vi "Estimate Time.vi"(8 "error in (no error)":errorcluster, 11 "Scan Driver in":refnum<class "Scan Driver.lvclass">) -> (0 "error out":errorcluster, 1 "Seconds":dbl[unit], 2 "Time Estimate":string, 3 "Scan Driver out":refnum<class "Scan Driver.lvclass">)   [LabVIEW 2009, in "Scan Driver.lvclass"]
doc: "Estimate the time needed to complete this Scan Driver instance, using data from member Scanner and Reader."
uses:
  Scan Driver.lvclass
  Scan Driver.lvclass/Scan Driver.ctl
  Readers/Reader/Reader.lvclass
  Scanners/Scanner/Scanner.lvclass
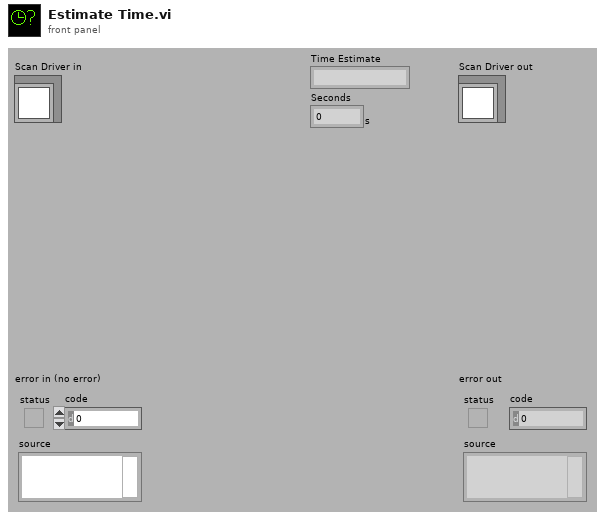
[diagram p1: front panel]
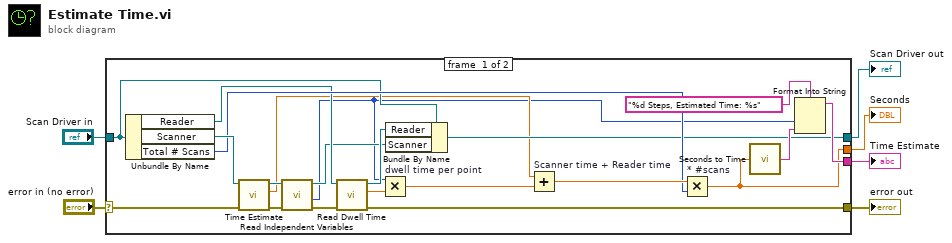
[diagram p0: block diagram]
diagram:
  n1 = case shown="No Error" "error in (no error)" {
    selector: "error in (no error)" -> [w10 w29]
    tunnel: [w23 _] -> w2
    tunnel: [w22 _] -> w1
    tunnel: [w14 w28] -> w5
    tunnel: [w8 w29] -> w6
    tunnel: "Scan Driver in" -> [w13 w28]
    frame #0 {
      n2 = Unbundle By Name(w13) -> ("Reader"=w18:refnum<class "Reader.lvclass">, "Scanner"=w21:refnum<class "Scanner.lvclass">, "Total # Scans"=w19:u32)
      n3 = call-dynamic "Time Estimate.vi"("error in (no error)"=w10, "Scanner.lvclass"=w21) -> ("error out"=w12:errorcluster, "time"=w11:dbl[unit], "Scanner.lvclass out"=w20:refnum<class "Scanner.lvclass">)  [unwired: 2 in, 5 out]
      n4 = call-dynamic "Read Independent Variables.vi"("error in (no error)"=w12, "Scanner.lvclass in"=w20) -> ("error out"=w9:errorcluster, "size"=w7:i32, "Scanner.lvclass out"=w15:refnum<class "Scanner.lvclass">)  [unwired: 7 out]
      n5 = call-dynamic "Read Dwell Time.vi"("error in (no error)"=w9, "Reader.lvclass in"=w18) -> ("error out"=w8:errorcluster, "Dwell Time"=w17:dbl[unit], "Reader.lvclass out"=w16:refnum<class "Reader.lvclass">)  [unwired: 7 out]
      n6 = Multiply "dwell time per point"(x=w7, y=w17) -> (x*y=w27:dbl[unit])
      n7 = Bundle By Name(cluster=w13, "Reader"=w16, "Scanner"=w15) -> (w14:refnum<class "Scan Driver.lvclass">)
      n8 = Add "Scanner time + Reader time"(x=w11, y=w27) -> (x+y=w26:dbl[unit])
      n9 = Multiply "* #scans"(x=w26, y=w19) -> (x*y=w22:dbl[unit])
      n10 = call "Seconds to Time.vi"("Seconds"=w22) -> ("Time"=w24:string)
      n11 = Format Into String(format string="%d Steps, Estimated Time: %s", w7, w24) -> (resulting string=w23:string)  [unwired: 2 in, 1 out]
    }
    frame #1 {
    }
  }
  "error out" <- w6
  "Scan Driver out" <- w5
  "Time Estimate" <- w2
  "Seconds" <- w1
